vi "FG-Frame-rate.vi"(8 "error in":errorcluster, 9 "Acquis. params. ref.":refnum<data-value>, 10 "Config file string in":string, 11 "Config. params. ref. in":refnum<data-value>) -> (0 "error IO":errorcluster, 1 "Number of replacements":i32, 2 "Config file string":string, 3 "Config. params. ref.":refnum<data-value>)   [LabVIEW 2013, in "CameraVision.lvlib" / "CV-Configuration.lvclass"]
uses:
  CV-Configuration.lvclass
  Acquisition/CV-Acquisition.lvclass
  CV-Configuration.lvclass/CV-Configuration.ctl
  Acquisition/CV-Acquisition.lvclass/CV-Acquisition.ctl
  Read Framegrabber DLL file.vi
  Read BoardHandle.vi
  Read Camport array.vi
  Acquisition/Read Maximum frame rate.vi
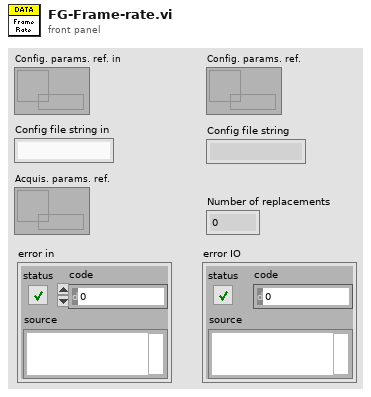
[diagram p1: front panel]
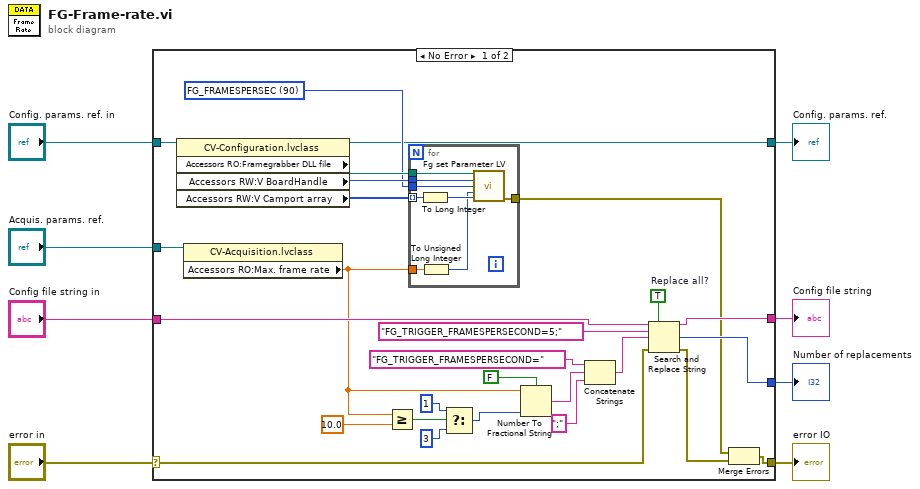
[diagram p0: block diagram]
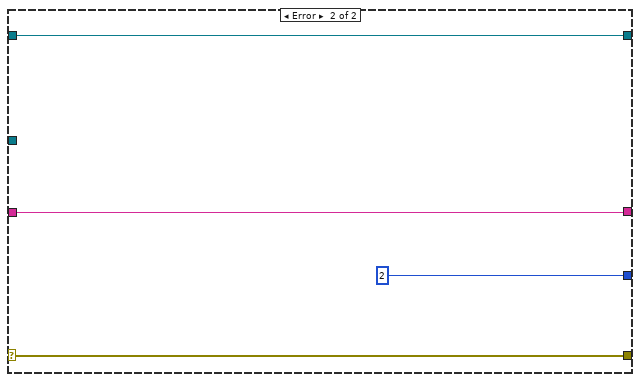
[diagram p2: hidden frame]
diagram:
  n1 = case shown="No Error" "error in" {
    selector: "error in" -> [w9 w45]
    tunnel: [w35 2 ("number of replacements")] -> w8
    tunnel: [w34 w47] -> w7
    tunnel: [w10 w45] -> w6
    tunnel: "Config file string in" -> [w33 w47]
    tunnel: "Acquis. params. ref." -> [w21 _]
    tunnel: "Config. params. ref. in" -> [w19 w44]
    tunnel: [w14 w44] -> w1
    frame No Error {
      w15 = 90 items=["FG_WIDTH"=100, "FG_HEIGHT"=200, "FG_FORMAT"=700, "FG_XOFFSET"=300, "FG_YOFFSET"=400, "FG_FRAMESPERSEC"=90, "FG_EXPOSURE"=10020, "FG_TRIGGERMODE"=8100, "FG_TRIGGERINSRC"=8110, "FG_TRIGGERSTATE"=300201, "FG_TRIGGER_LEGACY_MODE"=300254, "FG_CAMERA_LINK_CAMTYP"=11011, "FG_USEDVAL"=5025, "FG_SENSORREADOUT"=5050, "FG_STROBEPULSEDELAY"=8700, "FG_FLASH_POLARITY"=24060, "FG_EXSYNCINVERT"=8200, "FG_EXSYNCPOLARITY"=8420, "FG_EXSYNCDELAY"=8400, "FG_FLASHON"=8600, "FG_EXSYNCON"=8300, "FG_TRIGGERINPOLARITY"=8116, "FG_KNEE_LUT_FILE"=12110, "FG_KNEE_LUT_OFFSET"=12102, "FG_KNEE_LUT_SCALE"=12101, "FG_KNEE_LUT_GAMMA"=12103, "FG_KNEE_LUT_INVERT"=12104, "FG_CCSEL0"=14001, "FG_CCSEL1"=14002, "FG_CCSEL2"=14003, "FG_CCSEL3"=14004, "FG_DIGIO_OUTPUT"=14020, "FG_IMG_SELECT_PERIOD"=25110, "FG_IMG_SELECT"=25111, "FG_PORT"=3000, "FG_GLOBAL_ACCESS"=24110, "FG_TIMEOUT"=600] ("Ring")
      w20 = TRUE  # Replace all?
      n2 = property class="CV-Configuration.lvclass"(reference=w19) -> (reference out=w14:refnum<data-value>, "Accessors RO:Framegrabber DLL file"=w18:path, "Accessors RW:V BoardHandle"=w17:u64, "Accessors RW:V Camport array"=w16:u32[])  [unwired: 1 in, 1 out]
      n3 = property class="CV-Acquisition.lvclass"(reference=w21) -> ("Accessors RO:Max. frame rate"=w12:dbl)  [unwired: 1 in, 2 out]
      n4 = Greater Or Equal?(x=w12, y=10.0) -> (x >= y?=w25:bool)
      n5 = for {
        tunnel: w18 -> [w43]
        tunnel: w17 -> [w42]
        tunnel: w15 -> [w41]
        tunnel: w16 -> [w40] mode=indexing
        tunnel: w12 -> [w37]
        tunnel: [w38] -> w13
        n6 = To Long Integer(number=w40) -> (32bit integer=w39:i32)
        n7 = To Unsigned Long Integer(number=w37) -> (unsigned 32bit integer=w36:u32)
        n8 = call <userlib>:"Fg set Parameter LV.vi"("dll path in"=w43, "FgAddr"=w42, "Parameter"=w41, "Value"=w36, "CamPort"=w39) -> ("error out"=w38:errorcluster)  [unwired: 8 in, 2 out]
      }
      n9 = Select(t=i16 1 ("precision (6)"), s=w25, f=i16 3 ("precision (6)")) -> (s? t:f=w22:i16)
      n10 = Number To Fractional String(use system decimal point (T)=FALSE, number=w12, precision (6)=w22) -> (F-format string=w30:string)  [unwired: 1 in]
      n11 = Concatenate Strings("FG_TRIGGER_FRAMESPERSECOND=" ("search string"), w30, ";" ("string")) -> (w31:string)
      n12 = Search and Replace String(replace all?=w20, input string=w33, search string="FG_TRIGGER_FRAMESPERSECOND=5;", replace string=w31, error in=w9) -> (result string=w34:string, number of replacements=w35:i32, error out=w11:errorcluster)  [unwired: 3 in, 1 out]
      n13 = Merge Errors(w13, w11) -> (w10:errorcluster)
    }
    frame Error {
    }
  }
  "Number of replacements" <- w8
  "Config file string" <- w7
  "error IO" <- w6
  "Config. params. ref." <- w1
